vi "NewCountRate.vi"() -> ()   [LabVIEW 2014]
doc: "This VI counts the number of electrons per a time period by using a Gieger counter and then plots the data on a graph. The total time of the data aquisition and time interval is controlled by the user and the program runs and does a count till the time is over. Then it stores all the counts and writes the data to a spreadsheet."
uses:
  <vilib>/Platform/TimedLoop/XDataNode/timing_clust.ctl
  <vilib>/Platform/TimedLoop/XDataNode/nitl_modes.ctl
  <vilib>/Platform/TimedLoop/XDataNode/wakeup.ctl
  <vilib>/imath/engines/lvmath2/RunTimeEngine/Managers/WorkSpace/UID Generator.vi
  <vilib>/imath/engines/lvmath2/RunTimeEngine/BuiltInFunctions/linramp/NIMS_linramp.vi
  <vilib>/imath/engines/lvmath2/RunTimeEngine/RunTimeType/NIMS_RunTimeType_From StrictType (excl LVString).vi
  <instcachedir>/0/NIMS_RunTimeType_From StrictType (excl LVString)_15A5391EEA9C4AACB9955AC755B83D29.lvgen/NIMS_RunTimeType_From StrictType (excl LVString)_15A5391EEA9C4AACB9955AC755B83D29_000.vi
  <vilib>/imath/engines/lvmath2/RunTimeEngine/LocalVariableDefStatement/MC_LocalVariableDefStatement_Display.vi
  <vilib>/imath/engines/lvmath2/RunTimeEngine/Managers/SymbolTable/Clear UID.vi
  <vilib>/imath/engines/lvmath2/RunTimeEngine/NodeEndStatement/NIMS_NodeEndStatement_Output.vi
  <instcachedir>/0/NIMS_NodeEndStatement_Output_53EC0D466D134D7ABD903AC30B43404B.lvgen/NIMS_NodeEndStatement_Output_53EC0D466D134D7ABD903AC30B43404B_005.vi
  <vilib>/imath/engines/lvmath2/RunTimeEngine/ErrorHandling/NIMS_Finalize Error.vi
  <vilib>/Utility/file.llb/Write To Spreadsheet File (DBL).vi
  <vilib>/platform/TimedLoop/XDataNode/XDataNode.xnode
  <vilib>/Platform/TimedLoop/XDataNode/XDNodeRunTimeDep.lvlib
  <vilib>/imath/engines/lvmath2/RunTimeEngine/Managers/SymbolTable/NIMS_WorkSpace.lvlib
panel:
  in  "Path":path=path "U:/week8_new/run2_1secInt_5min"
  out "Waveform Graph":i32[](graph)=[0, 83, 82, 87, 85, 81, 83, 81, 74, 72, 62, 72, 82, 86, 74, 77, 65, 70, 75, 69, 75, 82, 71, 70, 67, 70, 49, 70, 68, 76, 67, 72, 64, 75, 80, 69, 73, 57, 60, 46, 64, 64, 64, 58, 61, 61, 61, 70, 61, 60, 60, 71, 60, 64, 63, 56, 58, 63, 52, 55, 52, 59, 53, 59, 42, 65, 42, 64, 56, 62, 49, 37, 47, 51, 40, 50, 41, 50, 40, 38, 33, 51, 40, 44, 34, 38, 59, 46, 36, 38, 46, 34, 34, 39, 43, 47, 32, 36, 30, 25, 34, 37, 36, 38, 24, 24, 31, 29, 39, 34, 29, 25, 21, 29, 25, 39, 36, 39, 25, 33, 33, 32, 24, 24, 28, 32, 30, 34, 25, 21, 21, 24, 17, 22, 27, 31, 18, 21, 18, 25, 25, 30, 21, 39, 29, 24, 23, 12, 21, 16, 31, 21, 19, 18, 20, 16, 24, 21, 10, 17, 21, 20, 18, 18, 16, 19, 16, 33, 26, 15, 15, 20, 15, 13, 14, 21, 12, 13, 16, 13, 16, 13, 10, 18, 23, 13, 14, 15, 16, 20, 12, 15, 18, 16, 14, 8, 9, 11, 11, 15, 15, 14, 13, 16, 13, 9, 14, 12, 11, 11, 14, 18, 8, 13, 6, 12, 12, 10, 8, 7, 17, 10, 11, 7, 13, 16, 15, 13, 9, 10, 16, 8, 11, 9, 12, 13, 8, 12, 8, 9, 5, 9, 7, 12, 13, 11, 12, 9, 7, 13, 12, 7, 6, 15, 9, 10, 7, 7, 10, 6, 14, 8, 5, 8, 13, 10, 13, 4, 7, 10, 11, 13, 7, 6, 8, 5, 6, 10, 8, 9, 10, 10, 6, 10, 4, 7, 6, 6, 5, 7, 9, 4, 9, 6, 6, 13, 6, 4, 7, 3, 7]
  in  "Total Collection Time (s)":dbl=300.0
  in  "Collection Period  (ms)":i64=1000
  out "Array":i32[](array[numeric])=[0, 83, 82, 87, 85, 81, 83, 81, 74, 72, 62, 72, 82, 86, 74, 77, 65, 70, 75, 69, 75, 82, 71, 70, 67, 70, 49, 70, 68, 76, 67, 72, 64, 75, 80, 69, 73, 57, 60, 46, 64, 64, 64, 58, 61, 61, 61, 70, 61, 60, 60, 71, 60, 64, 63, 56, 58, 63, 52, 55, 52, 59, 53, 59, 42, 65, 42, 64, 56, 62, 49, 37, 47, 51, 40, 50, 41, 50, 40, 38, 33, 51, 40, 44, 34, 38, 59, 46, 36, 38, 46, 34, 34, 39, 43, 47, 32, 36, 30, 25, 34, 37, 36, 38, 24, 24, 31, 29, 39, 34, 29, 25, 21, 29, 25, 39, 36, 39, 25, 33, 33, 32, 24, 24, 28, 32, 30, 34, 25, 21, 21, 24, 17, 22, 27, 31, 18, 21, 18, 25, 25, 30, 21, 39, 29, 24, 23, 12, 21, 16, 31, 21, 19, 18, 20, 16, 24, 21, 10, 17, 21, 20, 18, 18, 16, 19, 16, 33, 26, 15, 15, 20, 15, 13, 14, 21, 12, 13, 16, 13, 16, 13, 10, 18, 23, 13, 14, 15, 16, 20, 12, 15, 18, 16, 14, 8, 9, 11, 11, 15, 15, 14, 13, 16, 13, 9, 14, 12, 11, 11, 14, 18, 8, 13, 6, 12, 12, 10, 8, 7, 17, 10, 11, 7, 13, 16, 15, 13, 9, 10, 16, 8, 11, 9, 12, 13, 8, 12, 8, 9, 5, 9, 7, 12, 13, 11, 12, 9, 7, 13, 12, 7, 6, 15, 9, 10, 7, 7, 10, 6, 14, 8, 5, 8, 13, 10, 13, 4, 7, 10, 11, 13, 7, 6, 8, 5, 6, 10, 8, 9, 10, 10, 6, 10, 4, 7, 6, 6, 5, 7, 9, 4, 9, 6, 6, 13, 6, 4, 7, 3, 7]
  out "counts per second":dbl(knob)=7.0 scale=0.0..100.0
  # "Count Rate VI for Physics 434"
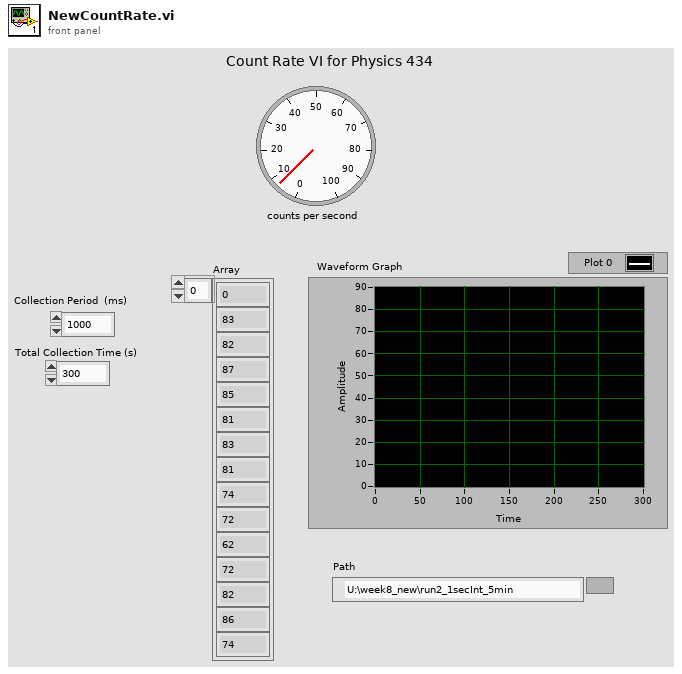
[diagram p1: front panel]
types:
  T1 = typedef "XDNodeRunTimeDep.lvlib/timing_clust.ctl" = cluster{"Expected End [f-1]":u64, "Actual End [f-1]":u64, "Finished Late? [f-1]":bool, "Expected End [i-1]":u64, "Actual End [i-1]":u64, "Finished Late? [i-1]":bool, "Expected Start [i]":u64, "Actual Start [i]":u64, "Expected Start [f]":u64, "Actual Start [f]":u64, "Source Name":string, "Structure Name":string, "Period":i64, "Deadline":i64, "Offset":i64, "Start":i64, "Priority":i32, "Timeout":i32, "Mode":T2, "Wakeup Reason":T3, "Error":errorcluster, "Source Type":string, "Secondary Source Type":string, "Global End Time":u64, "Global Start Time":u64, "Frame Duration":u64, "Iteration Duration":u64, "Assigned CPU":i32, "I/O Scan Engine Mode":u32}
  T2 = typedef "XDNodeRunTimeDep.lvlib/nitl_modes.ctl" = enum32{"No Change", "Process missed periods, maintain original phase", "Discard missed periods, maintain original phase", "Process missed periods, ignore original phase", "Discard missed periods, ignore original phase"}
  T3 = typedef "XDNodeRunTimeDep.lvlib/wakeup.ctl" = enum32{"Normal", "Aborted", "Asynchronous wakeup", "Timing source error", "Timed loop error", "Timeout"}
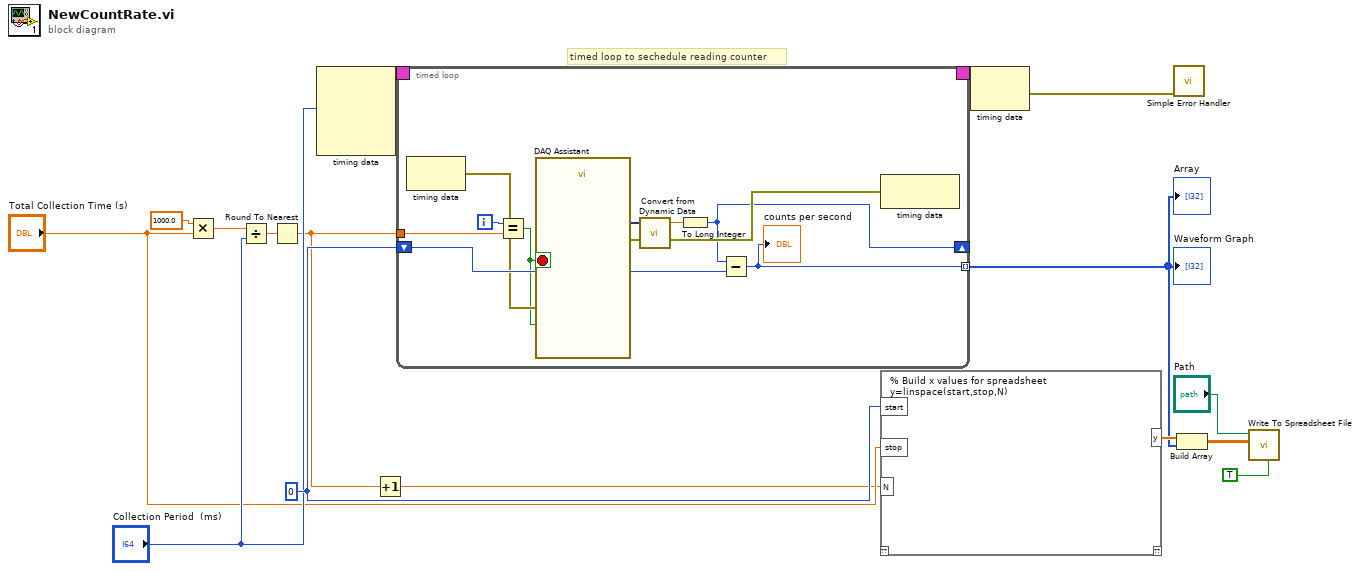
[diagram p0: block diagram]
diagram:
  w10 = 0
  # "timed loop to sechedule reading counter"
  n1 = Multiply(x=1000.0, y="Total Collection Time (s)") -> (x*y=w12:dbl)
  n2 = Divide(x=w12, y="Collection Period  (ms)") -> (x/y=w13:dbl)
  n3 = Round To Nearest(number=w13) -> (nearest integer value=w7:dbl)
  n4 = node-c288("Collection Period  (ms)") -> (w16:T1)  [unwired: 3 in]
  n5 = Increment(x=w7) -> (x+1=w6:dbl)
  n6 = timed-loop {
    timing: w16 -> [_]
    timing-out: [_] -> w15
    shift-right: [w21] -> _
    shift-left: w10 -> [w25]
    tunnel: [w20] -> w4 mode=indexing
    tunnel: w7 -> [w19]
    i -> [w18]
    stop <- w17 stop-if-true
    n7 = node-c288() -> (w22:errorcluster)  [unwired: 1 in]
    n8 = Equal?(x=w18, y=w19) -> (x = y?=w17:bool)
    n9 = call "DAQ Assistant"("error in"=w22, "stop (F)"=w17) -> ("data"=w26:dynamicdata, "error out"=w23:errorcluster)  [unwired: 14 in, 2 out]
    n10 = call "Convert from Dynamic Data"("Dynamic Data Type"=w26) -> ("Scalar"=w24:dbl)  [unwired: 3 in]
    n11 = To Long Integer(number=w24) -> (32bit integer=w21:i32)
    n12 = Subtract(x=w21, y=w25) -> (x-y=w20:i32)
    "counts per second" <- w20
    n13 = node-c288(w23) -> ()  [unwired: 1 out]
  }
  "Array" <- w4
  "Waveform Graph" <- w4
  n14 = mathscript code="% Build x values for spreadsheet\ny=linspace(start,stop,N)"("start"=w10, "stop"="Total Collection Time (s)", "N"=w6) -> ("y"=w5:dbl[])  [unwired: 1 in, 1 out]
  n15 = node-c288(w15) -> (w14:errorcluster)
  n16 = call <vilib>:"Simple Error Handler.vi"("error in (no error)"=w14) -> ()  [unwired: 4 in, 5 out]
  n17 = Build Array(w5, w4) -> (w3:dbl[][])
  n18 = call-poly <vilib>:"Write To Spreadsheet File.vi"("transpose? (no:F)"=TRUE, "2D data"=w3, "file path (dialog if empty)"="Path") -> ()  [unwired: 5 in, 1 out]
